vi "Write OVP_Enable.vi"(8 "error in":errorcluster, 10 "OVP_Enable":bool, 11 "57XX in":refnum<class "57XX.lvclass">) -> (0 "error out":errorcluster, 3 "57XX out":refnum<class "57XX.lvclass">)   [LabVIEW 2019, in "57XX.lvlib" / "57XX.lvclass"]
uses:
  Library/57XX.lvclass
  builds/Instruments/PowerSupply.lvlibp/Library/PowerSupply.lvclass
  builds/Engine/Engine.lvlibp/Project/Engine.lvclass
  C:/Users/Public/Documents/Development/builds/Engine/Engine.lvlibp/Project/Engine.lvclass
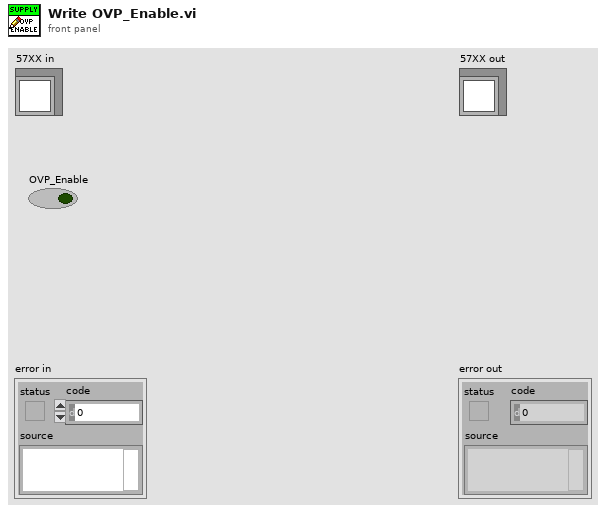
[diagram p1: front panel]
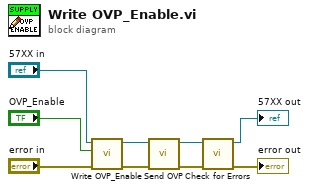
[diagram p0: block diagram]
diagram:
  n1 = call-parent "Write OVP_Enable.vi"("error in"="error in", "OVP_Enable"="OVP_Enable", "PowerSupply in"="57XX in") -> ("error out"=w5:errorcluster, "PowerSupply out"=w6:refnum<class "57XX.lvclass">)  [unwired: 7 in]
  n2 = call "Send OVP.vi"("error in (no error)"=w5, "57XX in"=w6) -> ("error out"=w4:errorcluster, "57XX out"=w2:refnum<class "57XX.lvclass">)  [unwired: 8 in]
  n3 = call "Check for Errors.vi"("error in"=w4, "Engine in"=w2) -> ("error out"=→"error out":errorcluster, "Engine out"=→"57XX out":refnum<class "57XX.lvclass">)  [unwired: 8 in]
